vi "TIFF Reader.vi"(10 "index":i32, 11 "Array":path[](array[path])) -> (3 "Image Out":T1)   [LabVIEW 2011]
uses:
  <vilib>/vision/Image Controls.llb/IMAQ Image.ctl
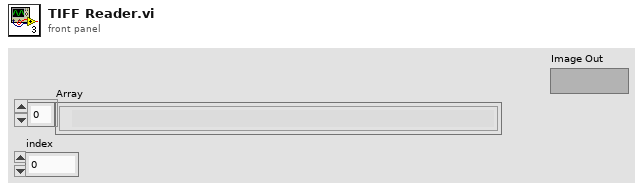
[diagram p1: front panel]
types:
  T1 = typedef "IMAQ Image.ctl" = refnum<image>
  T2 = typedef "Image Type" = u32
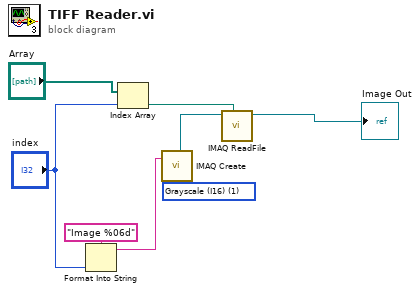
[diagram p0: block diagram]
diagram:
  w5 = T2 1 items=["Grayscale (U8)", "Grayscale (I16)", "Grayscale (SGL)", "Complex (CSG)", "RGB (U32)", "HSL (U32)", "RGB (U64)", "Grayscale (U16)"] ("Image Type")
  n1 = Format Into String(format string="Image %06d", "index") -> (resulting string=w2:string)  [unwired: 2 in, 1 out]
  n2 = Index Array(array="Array", index="index") -> (element=w7:path)
  n3 = call "IMAQ Create"("Image Name"=w2, "Image Type"=w5) -> ("New Image"=w6:T1)  [unwired: 3 in, 1 out]
  n4 = call "IMAQ ReadFile"("File Path"=w7, "Image"=w6) -> ("Image Out"=→"Image Out":T1)  [unwired: 5 in, 4 out]
